vi "Make ramp array.vi"(9 "step":dbl, 10 "end":dbl, 11 "start":dbl) -> (3 "Ramp Array":dbl[](array[numeric]))   [LabVIEW 2016]
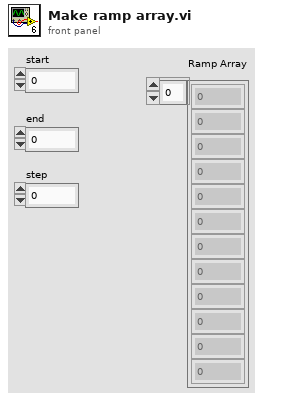
[diagram p1: front panel]
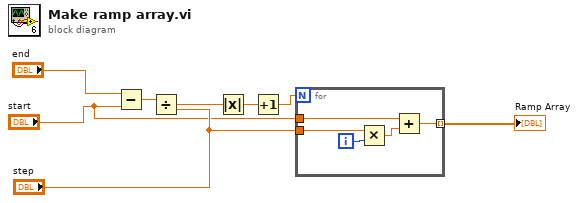
[diagram p0: block diagram]
diagram:
  n1 = Subtract(x="end", y="start") -> (x-y=w7:dbl)
  n2 = Divide(x=w7, y="step") -> (x/y=w8:dbl)
  n3 = Absolute Value(x=w8) -> (abs(x)=w1:dbl)
  n4 = Increment(x=w1) -> (x+1=w6:dbl)
  n5 = for {
    N: w6 -> [_]
    tunnel: "step" -> [w12]
    tunnel: "start" -> [w11]
    tunnel: [w9] -> w2 mode=indexing
    i -> [w13]
    n6 = Multiply(x=w12, y=w13) -> (x*y=w10:dbl)
    n7 = Add(x=w11, y=w10) -> (x+y=w9:dbl)
  }
  "Ramp Array" <- w2
